vi "Launcher Preparation.vi"(0 "Shooting Motors":dbl, 1 "Elevation":dbl, 2 "Set?":bool) -> (3 "Cannon":dbl, 4 "zAvit":dbl, 5 "Aim?":bool, 6 "Ready?":bool)   [LabVIEW 2012]
uses:
  BotStatus.vi
  <vilib>/express/express arith-compare/Formula/XNode/ExpressFormulaBlockNode.xnode
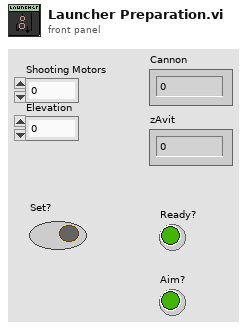
[diagram p1: front panel]
types:
  T1 = typedef "WPI_EncoderDevRef.ctl" = cluster{"DevStatus":errorcluster, "EncoderIndex":T2, "CounterIndex":T3, "DistancePerCount":dbl, "Decoding Type":T4}
  T2 = typedef "FPGA_EncoderIdx.ctl" = enum8{"Enc 0", "Enc 1", "Enc 2", "Enc 3", "Invalid"}
  T3 = typedef "FPGA_CounterCtrSystemIndex.ctl" = enum8{"Ctr 0", "Ctr 1", "Ctr 2", "Ctr 3", "Ctr 4", "Ctr 5", "Ctr 6", "Ctr 7", "Invalid"}
  T4 = typedef "WPI_EncoderType.ctl" = enum16{"1x", "2x", "4x"}
  T5 = cluster{"Middle":bool, "InCannon":bool, "InFlipper":bool, "FlipperAtPlace":bool, "Bottom":bool, "FrisbeeDirection":bool}
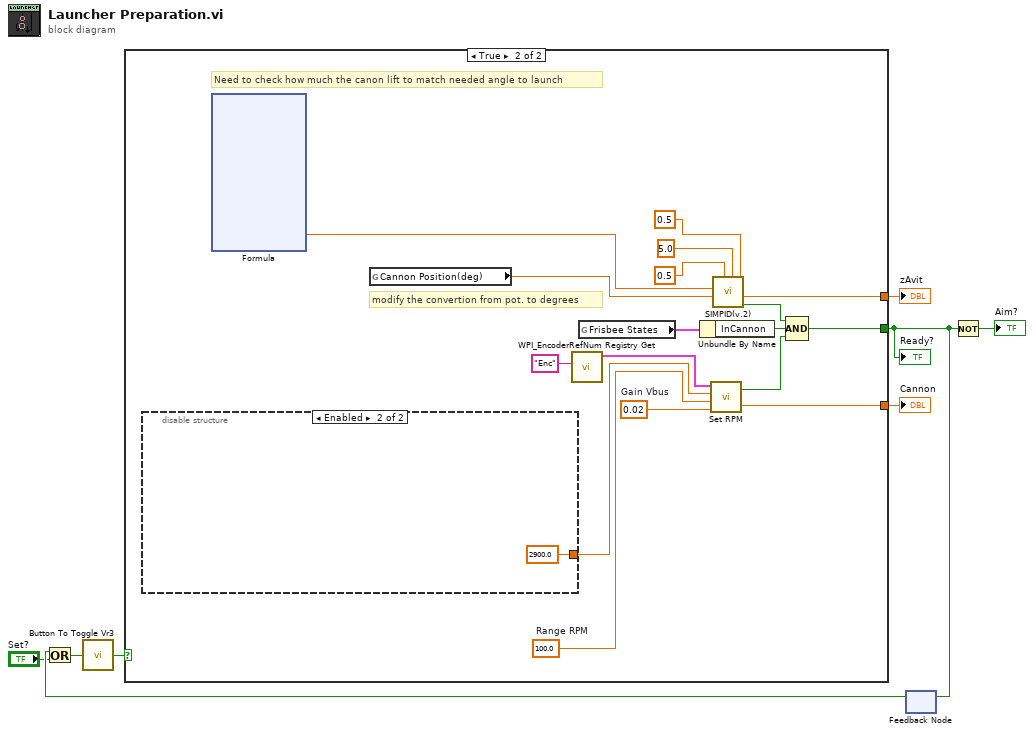
[diagram p0: block diagram]
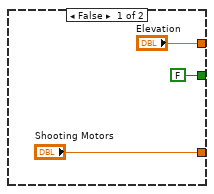
[diagram p2: hidden frame]
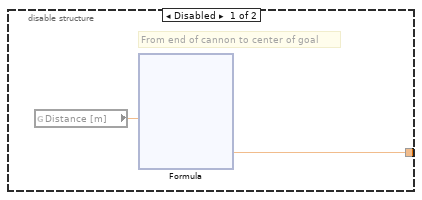
[diagram p3: hidden frame]
diagram:
  n1 = feedback #1() -> (w6:bool)  [unwired: 1 in]
  n2 = Or(x=w6, y="Set?") -> (x .or. y?=w8:bool)
  n3 = call "Button To Toggle Vr3.vi"("InValue"=w8) -> ("Result"=w7:bool)
  n4 = case shown="True" w7 {
    tunnel: ["Elevation" w24] -> w4
    tunnel: ["Shooting Motors" w22] -> w5
    tunnel: [FALSE w19] -> w1
    frame False {
    }
    frame True {
      w20 = 0.02  # Gain Vbus
      w21 = 100.0  # Range RPM
      # "modify the convertion from pot. to degrees"
      # "Need to check how much the canon lift to match needed angle to launch"
      n5 = disable-structure shown="Enabled" {
        disable-tunnel: [w29 2900.0 ("Set Point RPM")] -> w23
        frame Disabled {
          # "From end of cannon to center of goal"
          n6 = global read "BotStatus.vi" "Distance [m]"() -> (w30:dbl)
          n7 = xnode "Formula"("D"=w30) -> ("Result"=w29:dbl)  [unwired: 2 in, 1 out]
        }
        frame Enabled {
        }
      }
      n8 = xnode "Formula"() -> ("Result"=w12:dbl)  [unwired: 5 in, 1 out]
      n9 = global read "BotStatus.vi" "Cannon Position(deg)"() -> (w25:dbl)
      n10 = call <vilib>:"WPI_EncoderRefNum Registry Get.vi"("refnum name"="Enc") -> ("EncoderDevRef"=w18:T1)  [unwired: 9 in, 1 out]
      n11 = global read "BotStatus.vi" "Frisbee States"() -> (w16:T5)
      n12 = Unbundle By Name(w16) -> ("InCannon"=w13:bool)
      n13 = call "Set RPM.vi"("Gain Vbus"=w20, "Range RPM"=w21, "Set Point RPM"=w23, "EncoderDevRef"=w18) -> ("Vbus Out"=w22:dbl, "READY!"=w14:bool)
      n14 = call "SIMPID(v.2).vi"("Range"=0.5, "upper limit"=5.0, "lower limit"=0.5, "Current Point"=w25, "Set Point"=w12) -> ("On Target"=w15:bool, "result"=w24:dbl)  [unwired: 5 in]
      n15 = Compound Arithmetic op=AND(w15, w13, w14) -> (w19:bool)
    }
  }
  "Cannon" <- w5
  "zAvit" <- w4
  "Ready?" <- w1
  n16 = feedback-in #1(w1) -> ()
  n17 = Not(x=w1) -> (.not. x?=→"Aim?":bool)
